vi "Remove All Frames.vi"(8 "error in":errorcluster, 11 "Incoming/Outgoing Ref":T1 format="%.0x") -> (0 "error out":errorcluster, 3 "Incoming/Outgoing Ref out":T1 format="%.0x")   [LabVIEW 2020, in "Communication Bus Template Scripting.lvlib"]
uses:
  <vilib>/NI VeriStand/Custom Device API/Custom Device Item Ref.ctl
  Communication Bus Template Scripting.lvlib
  <vilib>/NI VeriStand/Custom Device API/Custom Device API.lvlib
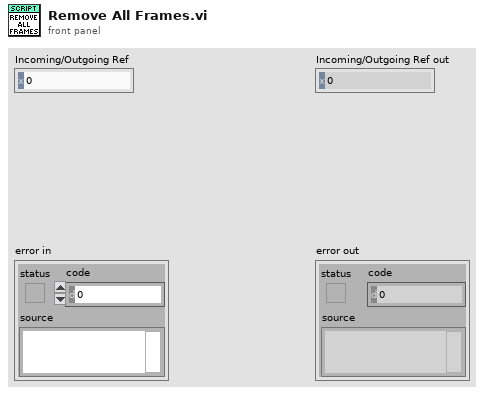
[diagram p1: front panel]
types:
  T1 = typedef "Custom Device API.lvlib/Custom Device Item Ref.ctl" = u64
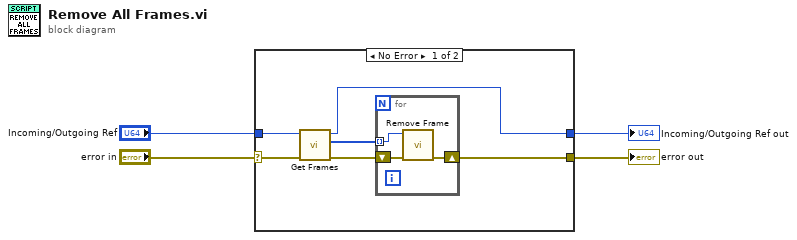
[diagram p0: block diagram]
diagram:
  n1 = case shown="No Error" "error in" {
    selector: "error in" -> [w8 w15]
    tunnel: "Incoming/Outgoing Ref" -> [w7 w14]
    tunnel: [w5 w15] -> w3
    tunnel: [w6 w14] -> w2
    frame No Error {
      n2 = call "Get Frames.vi"("error in"=w8, "Incoming/Outgoing in"=w7) -> ("error out"=w9:errorcluster, "Frames"=w10:T1[], "Incoming/Outgoing out"=w6:T1)  [unwired: 7 in]
      n3 = for {
        shift-right: [w12] -> w5
        shift-left: w9 -> [w13]
        tunnel: w10 -> [w11] mode=indexing
        n4 = call "Remove Frame.vi"("error in"=w13, "Frame Ref"=w11) -> ("error out"=w12:errorcluster)  [unwired: 9 in]
      }
    }
    frame Error {
    }
  }
  "error out" <- w3
  "Incoming/Outgoing Ref out" <- w2
